vi "Order JointState By Name.vi"(2 "JointState In":T1, 3 "Ordered Joint Names":string[](array[string])) -> (0 "all found?":bool, 1 "JointState Out":T1)   [LabVIEW 2013, in "Helpers.lvlib"]
uses:
  Helpers.lvlib
  labview_ros/sensor_msgs/JointState.ctl
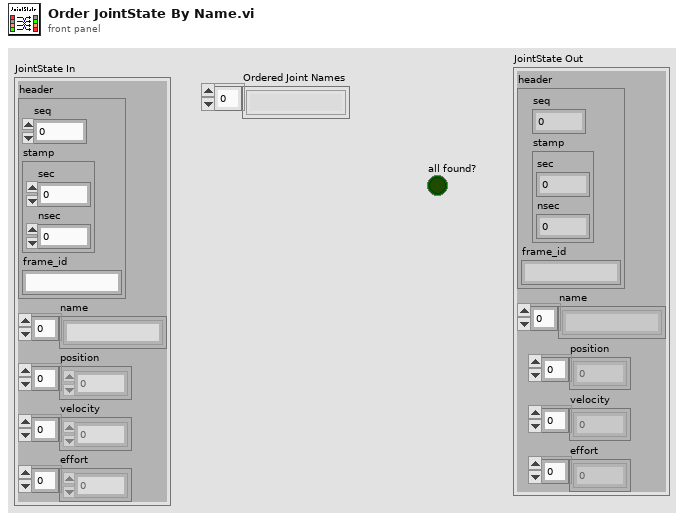
[diagram p1: front panel]
types:
  T1 = typedef "JointState.ctl" = cluster{"header":cluster{"seq":u32, "stamp":cluster{"sec":i32, "nsec":i32}, "frame_id":string}, "name":string[], "position":dbl[], "velocity":dbl[], "effort":dbl[]}
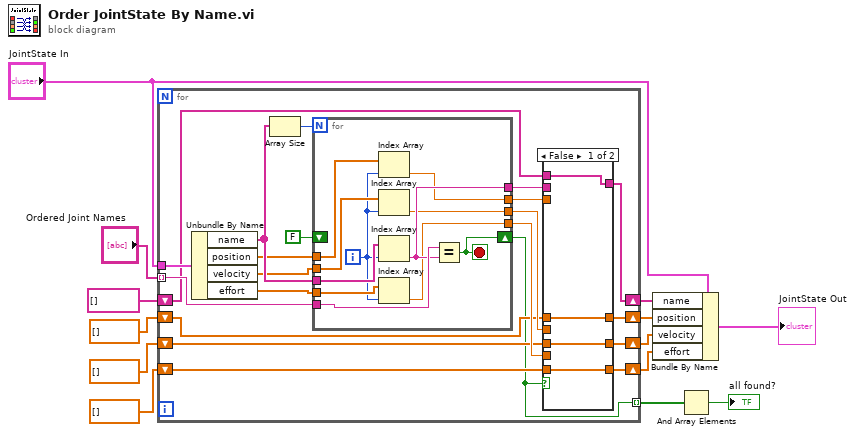
[diagram p0: block diagram]
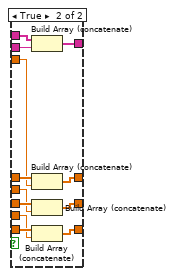
[diagram p2: hidden frame]
diagram:
  n1 = for {
    tunnel: "JointState In" -> [w34]
    tunnel: "Ordered Joint Names" -> [w31] mode=indexing
    shift-right: [w16] -> w5
    shift-left: dbl[] [] -> [w15]
    shift-right: [w18] -> w6
    shift-left: dbl[] [] -> [w17]
    shift-right: [w20] -> w7
    shift-left: dbl[] [] -> [w19]
    shift-right: [w22] -> w8
    shift-left: string[] [] -> [w21]
    tunnel: [w14] -> w2 mode=indexing
    n2 = Unbundle By Name(w34) -> ("name"=w32:string[], "position"=w30:dbl[], "velocity"=w29:dbl[], "effort"=w28:dbl[])
    n3 = Array Size(array=w32) -> (size(s)=w33:i32)
    n4 = for {
      N: w33 -> [_]
      tunnel: w32 -> [w61]
      tunnel: w31 -> [w60]
      tunnel: w30 -> [w59]
      tunnel: w29 -> [w58]
      tunnel: w28 -> [w57]
      tunnel: [w55] -> w26
      tunnel: [w54] -> w25
      tunnel: [w53] -> w24
      tunnel: [w52] -> w23
      shift-right: [w51] -> w14
      shift-left: FALSE -> [_]
      i -> [w56]
      stop <- w51 stop-if-true
      n5 = Index Array(array=w59, index=w56) -> (element=w54:dbl)
      n6 = Index Array(array=w58, index=w56) -> (element=w53:dbl)
      n7 = Index Array(array=w61, index=w56) -> (element=w55:string)
      n8 = Index Array(array=w57, index=w56) -> (element=w52:dbl)
      n9 = Equal?(x=w60, y=w55) -> (x = y?=w51:bool)
    }
    n10 = case shown="False" w14 {
      tunnel: w26 -> [_ w48]
      tunnel: w25 -> [_ w45]
      tunnel: w24 -> [_ w42]
      tunnel: w23 -> [_ w39]
      tunnel: [w38 w50] -> w22
      tunnel: w21 -> [w38 w49]
      tunnel: [w37 w47] -> w20
      tunnel: w19 -> [w37 w46]
      tunnel: [w36 w44] -> w18
      tunnel: w17 -> [w36 w43]
      tunnel: [w35 w41] -> w16
      tunnel: w15 -> [w35 w40]
      frame False {
      }
      frame True {
        n11 = Build Array (concatenate)(w49, w48) -> (w50:string[])
        n12 = Build Array (concatenate)(w46, w45) -> (w47:dbl[])
        n13 = Build Array (concatenate)(w43, w42) -> (w44:dbl[])
        n14 = Build Array (concatenate)(w40, w39) -> (w41:dbl[])
      }
    }
  }
  n15 = Bundle By Name(cluster="JointState In", "name"=w8, "position"=w7, "velocity"=w6, "effort"=w5) -> (→"JointState Out":T1)
  n16 = And Array Elements(Boolean array=w2) -> (logical AND=→"all found?":bool)
